vi "Counting Digital Numbers.vi"() -> ()   [LabVIEW 2021]
panel:
  out "Boolean 5":bool
  out "Boolean 4":bool
  out "Boolean 7":bool
  out "Boolean 6":bool
  out "Boolean 3":bool
  out "Boolean 2":bool
  out "Boolean":bool
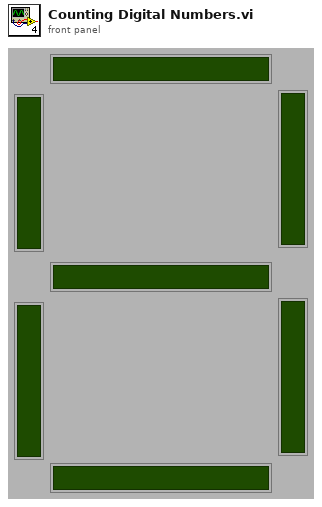
[diagram p1: front panel]
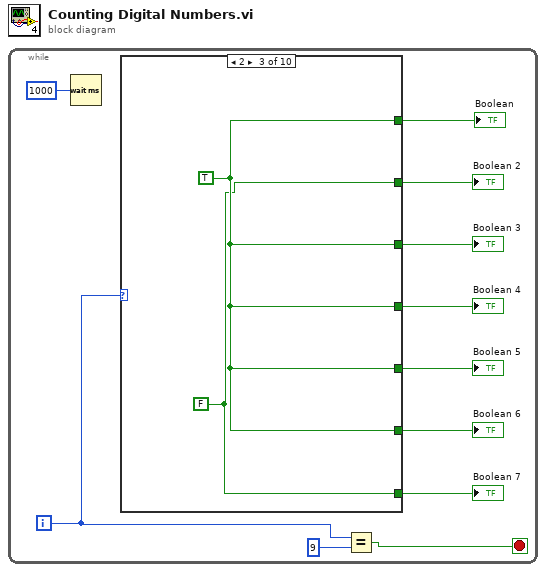
[diagram p0: block diagram]
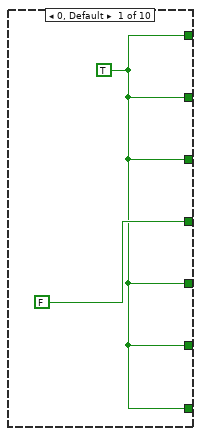
[diagram p2: hidden frame]
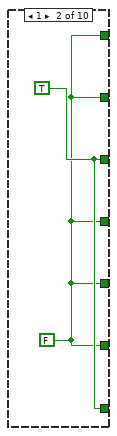
[diagram p3: hidden frame]
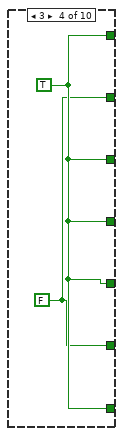
[diagram p4: hidden frame]
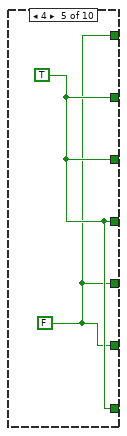
[diagram p5: hidden frame]
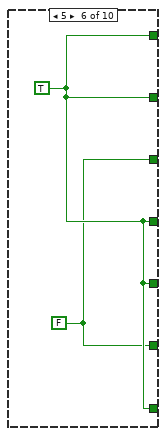
[diagram p6: hidden frame]
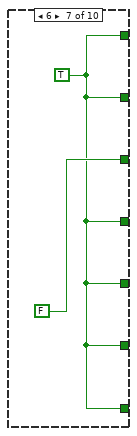
[diagram p7: hidden frame]
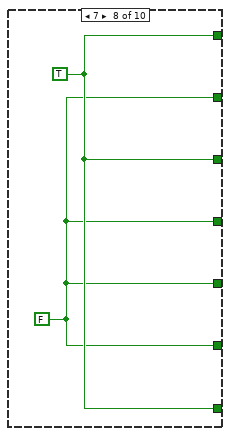
[diagram p8: hidden frame]
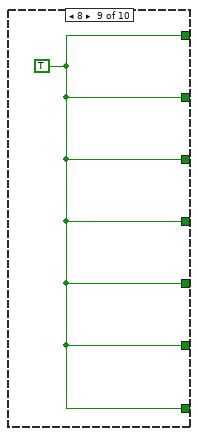
[diagram p9: hidden frame]
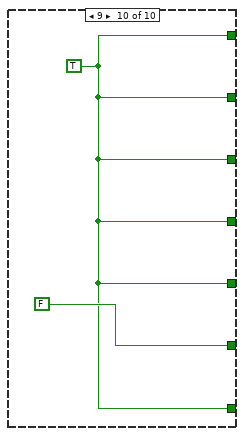
[diagram p10: hidden frame]
diagram:
  n1 = while {
    i -> [w10]
    stop <- w11 stop-if-true
    n2 = Wait (ms)(milliseconds to wait=u32 1000) -> ()  [unwired: 1 out]
    n3 = case shown="2" w10 {
      tunnel: [w12 w14 w17 w19 w20 w23 w24 w27 w28 w29] -> w8
      tunnel: [w12 w14 w16 w18 w21 w23 w24 w26 w28 w29] -> w7
      tunnel: [w12 w15 w17 w19 w21 w22 FALSE w27 w28 w29] -> w6
      tunnel: [FALSE w14 w17 w19 w21 w23 w24 w26 w28 w29] -> w5
      tunnel: [w12 w14 w17 w19 w20 w23 w24 w26 w28 w29] -> w4
      tunnel: [w12 w14 w17 w18 w20 w22 w24 w26 w28 FALSE] -> w3
      tunnel: [w12 w15 w16 w19 w21 w23 w24 w27 w28 w29] -> w2
      frame 0, Default {
        w12 = TRUE
      }
      frame 1 {
        w14 = FALSE
        w15 = TRUE
      }
      frame 2 {
        w16 = FALSE
        w17 = TRUE
      }
      frame 3 {
        w18 = FALSE
        w19 = TRUE
      }
      frame 4 {
        w20 = FALSE
        w21 = TRUE
      }
      frame 5 {
        w22 = FALSE
        w23 = TRUE
      }
      frame 6 {
        w24 = TRUE
      }
      frame 7 {
        w26 = FALSE
        w27 = TRUE
      }
      frame 8 {
        w28 = TRUE
      }
      frame 9 {
        w29 = TRUE
      }
    }
    "Boolean" <- w8
    "Boolean 2" <- w7
    "Boolean 3" <- w6
    "Boolean 6" <- w3
    "Boolean 7" <- w2
    "Boolean 4" <- w5
    "Boolean 5" <- w4
    n4 = Equal?(x=w10, y=9) -> (x = y?=w11:bool)
  }
